vi "PicoLogStart_3.vi"(0 "Ch nr":bool[](array[boolean]), 2 "Single ended\n(0- single)\n(1 - difer)":i32[](array[numeric]) min=0 max=1 step=1, 3 "sampleInterval_ms":i32=1000, 4 "Voltage range":i32[](array[numeric]) min=0 max=6 step=1, 6 "conversionTime":i16(ring) items=["60 ms", "100 ms", "180 ms", "340 ms", "660 ms"], 7 "Mains Frequency":i16(ring) items=["50 Hz", "60 Hz"]) -> (1 "Voltage range":i32[](array[numeric]), 5 "noOfChannels":i16=2, 8 "ChNrSkArr":i32[](array[numeric]), 9 "handle":i16, 10 "STOP":bool)   [LabVIEW 2014]
uses:
  Instance           1 22Saved   HRDL_streaming .vi
  Instance         138 22Saved   HRDL_streaming .vi
  picohrdl.dll
panel:
  out "Unit Info":T1
  # "1       2       3      4       5        6       7       8       9      10     11      12     13    14       15     16"
  # "0 -+2500mV\n1 -+1250mV\n2 -+625mV\n3 -+313mV\n4 -+156mV\n5 -+78mv\n6 -+39mV"
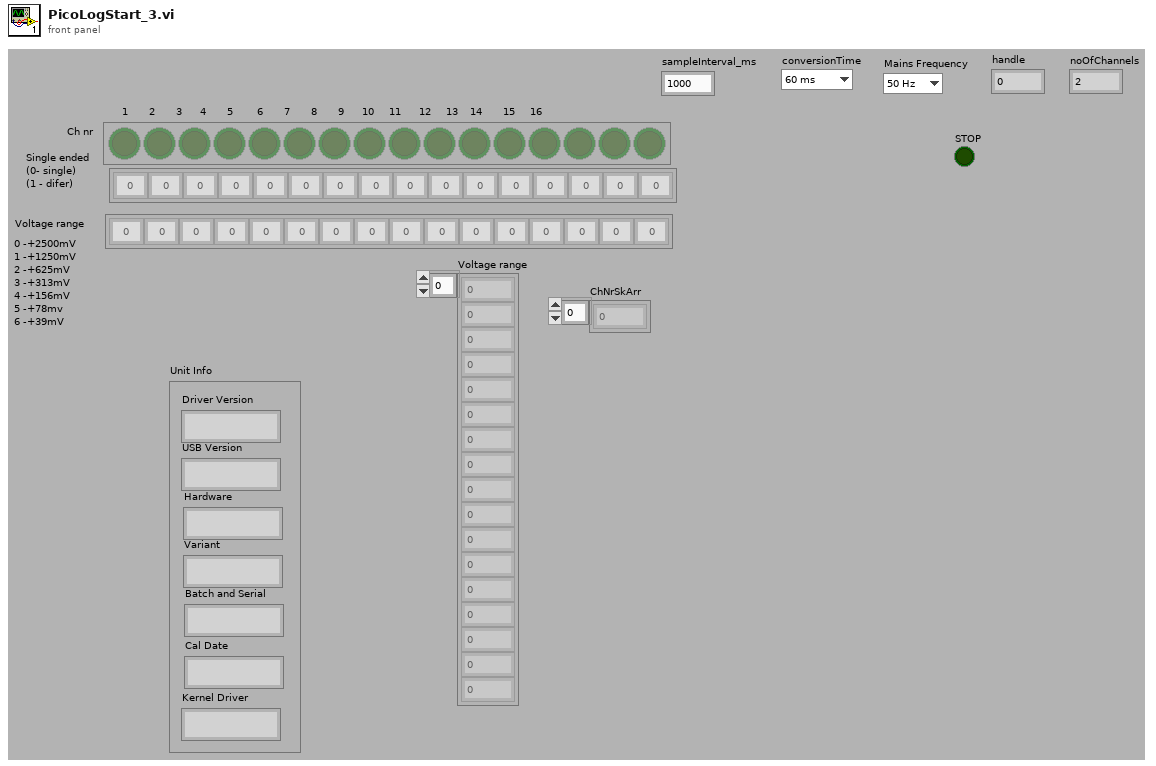
[diagram p1: front panel]
types:
  T1 = cluster{"Driver Version":string, "USB Version":string, "Hardware":string, "Variant":string, "Batch and Serial":string, "Cal Date":string, "Kernel Driver":string}
  T2 = cluster{"[0]":string, "[1]":string, "[2]":string, "[3]":string, "[4]":string, "[5]":string, "[6]":string}
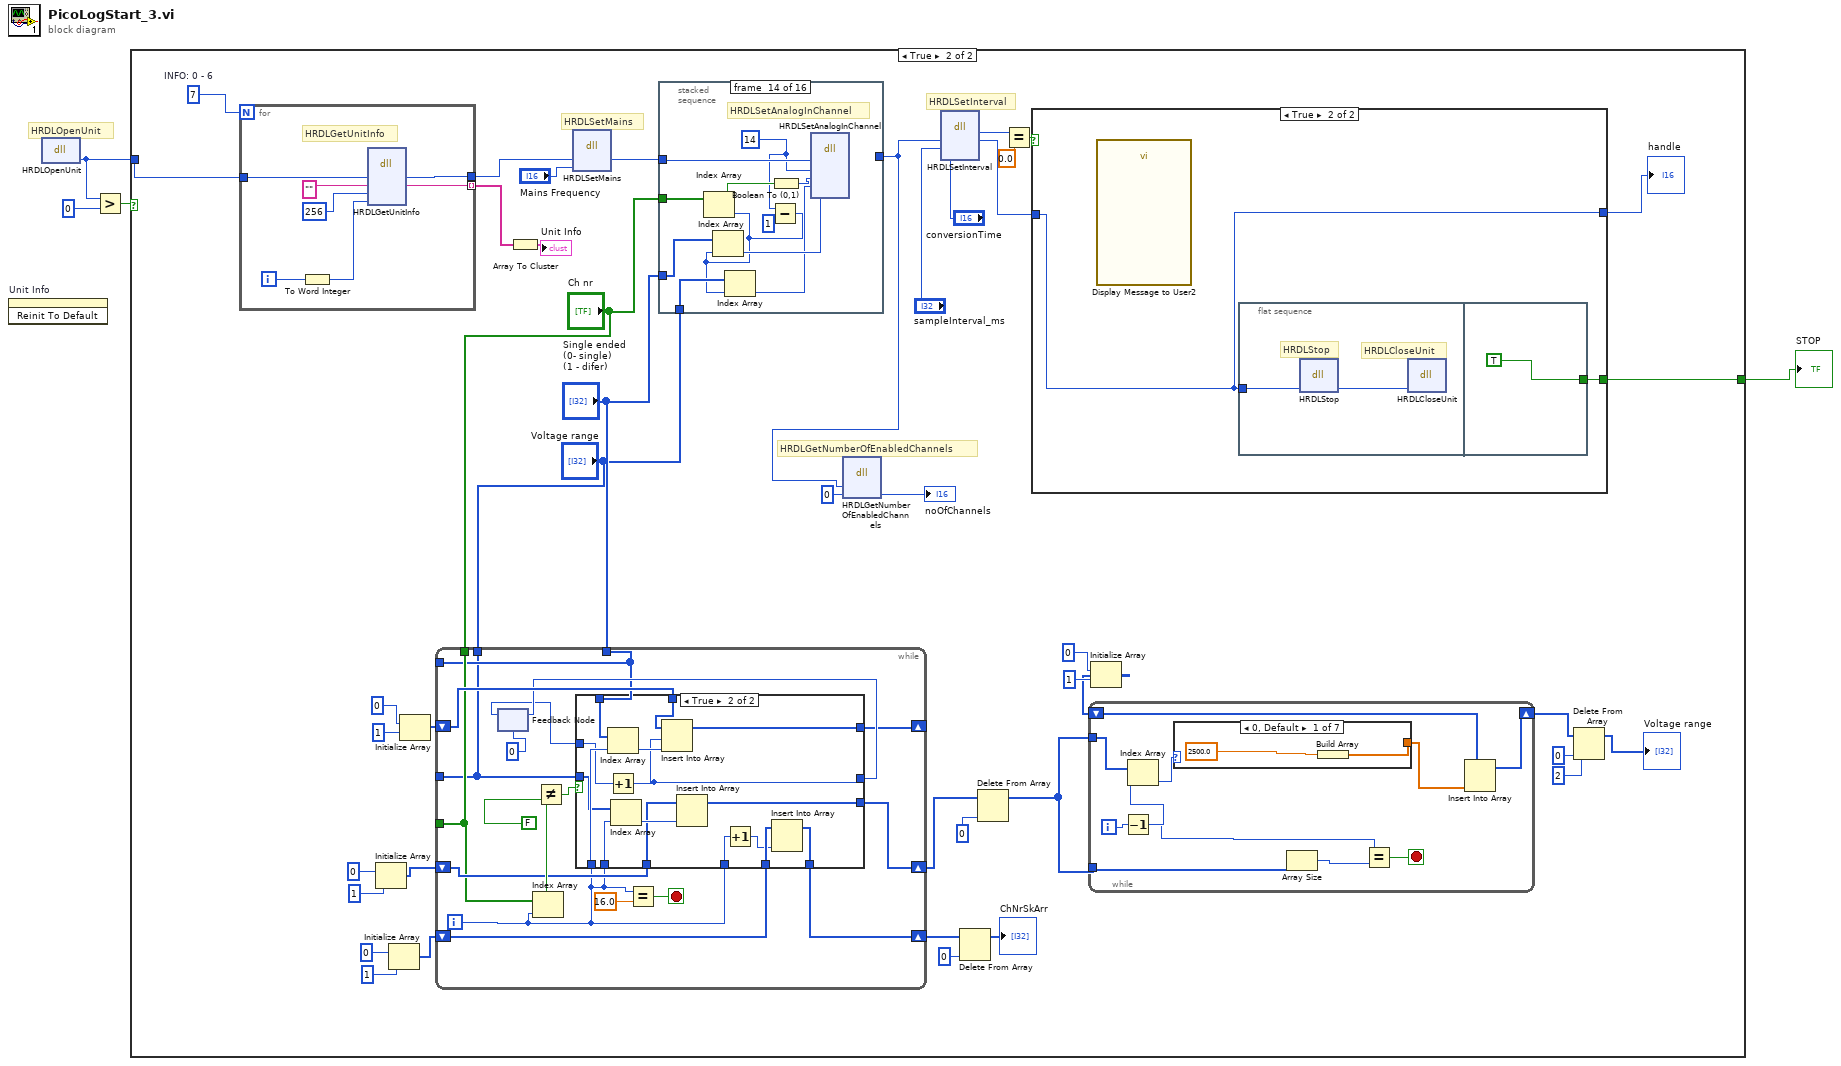
[diagram p0: block diagram]
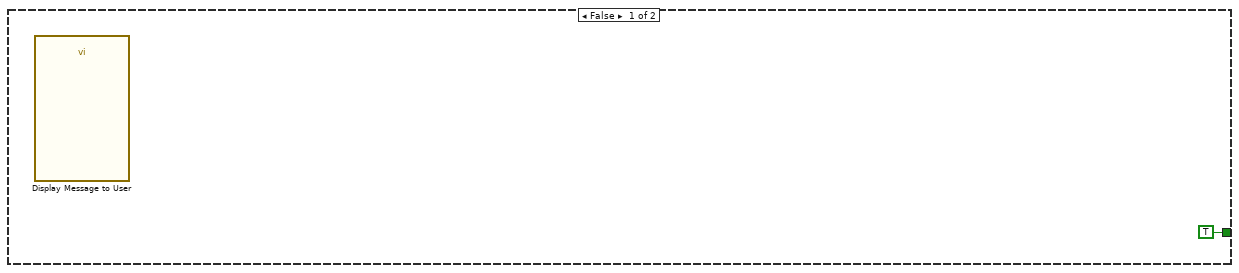
[diagram p2: hidden frame]
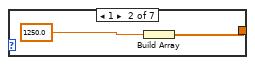
[diagram p3: hidden frame]
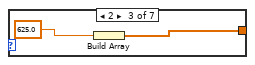
[diagram p4: hidden frame]
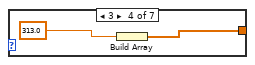
[diagram p5: hidden frame]
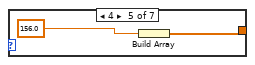
[diagram p6: hidden frame]
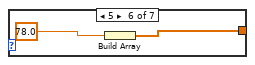
[diagram p7: hidden frame]
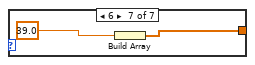
[diagram p8: hidden frame]
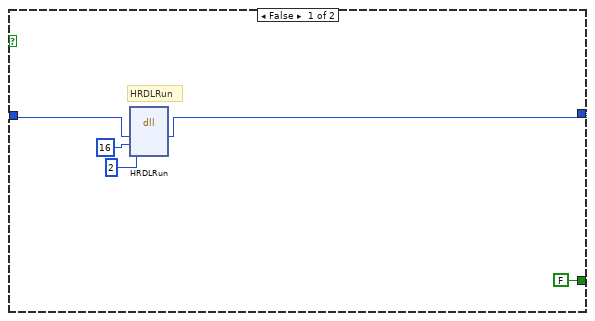
[diagram p10: hidden frame]
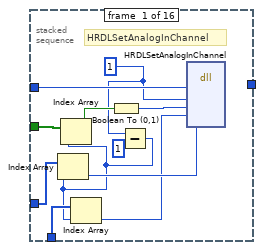
[diagram p11: hidden frame]
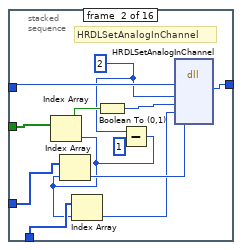
[diagram p12: hidden frame]
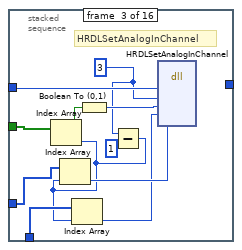
[diagram p13: hidden frame]
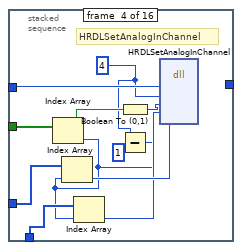
[diagram p14: hidden frame]
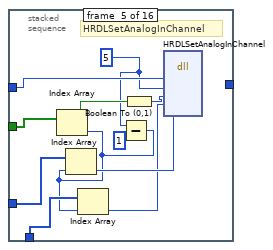
[diagram p15: hidden frame]
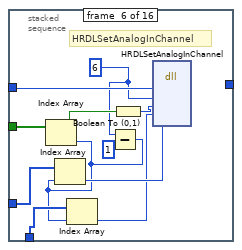
[diagram p16: hidden frame]
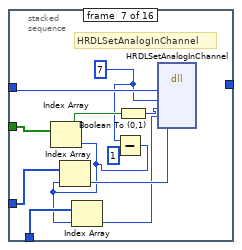
[diagram p17: hidden frame]
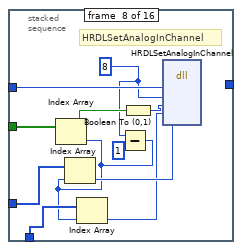
[diagram p18: hidden frame]
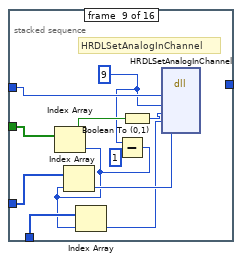
[diagram p19: hidden frame]
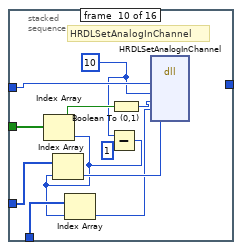
[diagram p20: hidden frame]
diagram:
  # "HRDLOpenUnit"
  n1 = invoke on="Unit Info" class="Clust (strict)" method="Reinit To Default"() -> ()  [unwired: 3 in, 3 out]
  n2 = dll-call lib="picohrdl.dll" fn="HRDLOpenUnit"() -> ("handle"=w2:i16)  [unwired: 3 in, 2 out]
  n3 = Greater?(x=w2, y=i16 0) -> (0:w4:bool)
  n4 = case shown="True" w4 {
    tunnel: w2 -> [_ w39]
    tunnel: [TRUE ("stop") w33] -> w1
    frame False {
      n5 = call "Display Message to User"() -> ()  [unwired: 10 in, 2 out]
    }
    frame True {
      w41 = 7  # INFO: 0 - 6
      # "HRDLGetNumberOfEnabledChannels"
      # "HRDLSetInterval"
      # "HRDLSetMains"
      n6 = for {
        N: w41 -> [_]
        tunnel: w39 -> [w117]
        tunnel: [w114] -> w38 mode=indexing
        tunnel: [w112] -> w40
        i -> [w113]
        # "HRDLGetUnitInfo"
        n7 = To Word Integer(number=w113) -> (16bit integer=w111:i16)
        n8 = dll-call lib="picohrdl.dll" fn="HRDLGetUnitInfo"("handle"=w117, "unitInfo"="", "stringLength"=i16 256, "info"=w111) -> ("handle"=w112:i16, "unitInfo"=w114:string)  [unwired: 6 in, 2 out]
      }
      n9 = Initialize Array(0 ("element"), 1 ("dimension size")) -> (w28:i32[])
      n10 = Initialize Array(0 ("element"), 1 ("dimension size")) -> (w9:i32[])
      n11 = Initialize Array(0 ("element"), 1 ("dimension size")) -> (w25:i32[])
      n12 = while {
        tunnel: [w78] -> _
        tunnel: [w77] -> _
        tunnel: [w76] -> _
        shift-right: [w82] -> w23
        shift-left: w28 -> [w81]
        shift-right: [w80] -> _
        shift-left: w25 -> [w87]
        tunnel: "Ch nr" -> [w78]
        tunnel: "Single ended\n(0- single)\n(1 - difer)" -> [w77]
        tunnel: "Voltage range" -> [w76]
        shift-right: [w73] -> w8
        shift-left: w9 -> [w75]
        i -> [w74]
        stop <- w83 stop-if-true
        n13 = feedback #1(i16 0 ("handle")) -> (w79:i16)
        n14 = Index Array(array=w78, index=w74) -> (element=w90:bool)
        n15 = Not Equal?(x=w90, y=FALSE) -> (x != y?=w88:bool)
        n16 = case shown="True" w88 {
          tunnel: w77 -> [_ w109]
          tunnel: w74 -> [_ w110]
          tunnel: w87 -> [w92 w107]
          tunnel: w79 -> [w94 w106]
          tunnel: [w94 w102] -> w85
          tunnel: w74 -> [_ w105]
          tunnel: w76 -> [_ w104]
          tunnel: [w93 w101] -> w82
          tunnel: w81 -> [w93 w100]
          tunnel: [w92 w99] -> w80
          tunnel: w75 -> [w91 w98]
          tunnel: w74 -> [_ w96]
          tunnel: [w91 w95] -> w73
          frame False {
          }
          frame True {
            n17 = Index Array(array=w109, index=w110) -> (element=w108:i32)
            n18 = Increment(x=w106) -> (x+1=w102:i16)
            n19 = Index Array(array=w104, index=w105) -> (element=w103:i32)
            n20 = Insert Into Array(array=w107, index=w102, new element=w108) -> (w99:i32[])
            n21 = Insert Into Array(array=w100, new element=w103) -> (w101:i32[])  [unwired: 1 in]
            n22 = Increment(x=w96) -> (x+1=w97:i32)
            n23 = Insert Into Array(array=w98, new element=w97) -> (w95:i32[])  [unwired: 1 in]
          }
        }
        n24 = feedback-in #1(w85) -> ()
        n25 = Equal?(x=w74, y=16.0) -> (x = y?=w83:bool)
      }
      n26 = Array To Cluster(array=w38) -> (cluster=→"Unit Info":T2)
      n27 = dll-call lib="PicoHRDL.dll" fn="HRDLSetMains"("handle"=w40, "sixtyHertz"="Mains Frequency") -> ("handle"=w32:i16)  [unwired: 5 in, 2 out]
      n28 = stacked-sequence {
        tunnel: w32 -> [w138 w146 w157 w165 w179 w190 w201 w212 w223 w234 w245 w256 w267 w278 w289 w300]
        tunnel: "Ch nr" -> [w136 w145 w156 w168 w178 w189 w200 w211 w222 w233 w244 w255 w266 w277 w288 w299]
        tunnel: "Single ended\n(0- single)\n(1 - difer)" -> [w134 w144 w155 w166 w177 w188 w199 w210 w221 w232 w243 w254 w265 w276 w287 w298]
        tunnel: "Voltage range" -> [w132 w143 w154 w167 w176 w187 w198 w209 w220 w231 w242 w253 w264 w275 w286 w297]
        tunnel: [_ w139 _ _ _ _ _ _ _ _ _ _ _ _ _ _] -> w31
        frame #0 {
          w130 = i16 1 ("channel")
          # "HRDLSetAnalogInChannel"
          n29 = Subtract(x=w130, y=i16 1) -> (x-y=w129:i16)
          n30 = Index Array(array=w134, index=w129) -> (element=w133:i32)
          n31 = Index Array(array=w136, index=w129) -> (element=w135:bool)
          n32 = Index Array(array=w132, index=w129) -> (element=w131:i32)
          n33 = Boolean To (0,1)(Boolean=w135) -> (0, 1=w137:i16)
          n34 = dll-call lib="PicoHRDL.dll" fn="HRDLSetAnalogInChannel"("handle"=w138, "channel"=w130, "enabled"=w137, "range"=w131, "singleEnded"=w133) -> ()  [unwired: 9 in, 2 out]
        }
        frame #1 {
          w141 = i16 2 ("channel")
          # "HRDLSetAnalogInChannel"
          n35 = Subtract(x=w141, y=i16 1) -> (x-y=w140:i16)
          n36 = Index Array(array=w145, index=w140) -> (element=w149:bool)
          n37 = Index Array(array=w144, index=w140) -> (element=w148:i32)
          n38 = Index Array(array=w143, index=w140) -> (element=w147:i32)
          n39 = Boolean To (0,1)(Boolean=w149) -> (0, 1=w150:i16)
          n40 = dll-call lib="PicoHRDL.dll" fn="HRDLSetAnalogInChannel"("handle"=w146, "channel"=w141, "enabled"=w150, "range"=w147, "singleEnded"=w148) -> ("handle"=w139:i16)  [unwired: 8 in, 2 out]
        }
        frame #2 {
          w152 = i16 3 ("channel")
          # "HRDLSetAnalogInChannel"
          n41 = Subtract(x=w152, y=i16 1) -> (x-y=w151:i16)
          n42 = Index Array(array=w156, index=w151) -> (element=w160:bool)
          n43 = Index Array(array=w155, index=w151) -> (element=w159:i32)
          n44 = Index Array(array=w154, index=w151) -> (element=w158:i32)
          n45 = Boolean To (0,1)(Boolean=w160) -> (0, 1=w161:i16)
          n46 = dll-call lib="PicoHRDL.dll" fn="HRDLSetAnalogInChannel"("handle"=w157, "channel"=w152, "enabled"=w161, "range"=w158, "singleEnded"=w159) -> ()  [unwired: 9 in, 2 out]
        }
        frame #3 {
          w163 = i16 4 ("channel")
          # "HRDLSetAnalogInChannel"
          n47 = Subtract(x=w163, y=i16 1) -> (x-y=w162:i16)
          n48 = Index Array(array=w168, index=w162) -> (element=w171:bool)
          n49 = Index Array(array=w166, index=w162) -> (element=w170:i32)
          n50 = Index Array(array=w167, index=w162) -> (element=w169:i32)
          n51 = Boolean To (0,1)(Boolean=w171) -> (0, 1=w172:i16)
          n52 = dll-call lib="PicoHRDL.dll" fn="HRDLSetAnalogInChannel"("handle"=w165, "channel"=w163, "enabled"=w172, "range"=w169, "singleEnded"=w170) -> ()  [unwired: 9 in, 2 out]
        }
        frame #4 {
          w174 = i16 5 ("channel")
          # "HRDLSetAnalogInChannel"
          n53 = Subtract(x=w174, y=i16 1) -> (x-y=w173:i16)
          n54 = Index Array(array=w178, index=w173) -> (element=w182:bool)
          n55 = Index Array(array=w177, index=w173) -> (element=w181:i32)
          n56 = Index Array(array=w176, index=w173) -> (element=w180:i32)
          n57 = Boolean To (0,1)(Boolean=w182) -> (0, 1=w183:i16)
          n58 = dll-call lib="PicoHRDL.dll" fn="HRDLSetAnalogInChannel"("handle"=w179, "channel"=w174, "enabled"=w183, "range"=w180, "singleEnded"=w181) -> ()  [unwired: 9 in, 2 out]
        }
        frame #5 {
          w185 = i16 6 ("channel")
          # "HRDLSetAnalogInChannel"
          n59 = Subtract(x=w185, y=i16 1) -> (x-y=w184:i16)
          n60 = Index Array(array=w189, index=w184) -> (element=w193:bool)
          n61 = Index Array(array=w188, index=w184) -> (element=w192:i32)
          n62 = Index Array(array=w187, index=w184) -> (element=w191:i32)
          n63 = Boolean To (0,1)(Boolean=w193) -> (0, 1=w194:i16)
          n64 = dll-call lib="PicoHRDL.dll" fn="HRDLSetAnalogInChannel"("handle"=w190, "channel"=w185, "enabled"=w194, "range"=w191, "singleEnded"=w192) -> ()  [unwired: 9 in, 2 out]
        }
        frame #6 {
          w196 = i16 7 ("channel")
          # "HRDLSetAnalogInChannel"
          n65 = Subtract(x=w196, y=i16 1) -> (x-y=w195:i16)
          n66 = Index Array(array=w200, index=w195) -> (element=w204:bool)
          n67 = Index Array(array=w199, index=w195) -> (element=w203:i32)
          n68 = Index Array(array=w198, index=w195) -> (element=w202:i32)
          n69 = Boolean To (0,1)(Boolean=w204) -> (0, 1=w205:i16)
          n70 = dll-call lib="PicoHRDL.dll" fn="HRDLSetAnalogInChannel"("handle"=w201, "channel"=w196, "enabled"=w205, "range"=w202, "singleEnded"=w203) -> ()  [unwired: 9 in, 2 out]
        }
        frame #7 {
          w207 = i16 8 ("channel")
          # "HRDLSetAnalogInChannel"
          n71 = Subtract(x=w207, y=i16 1) -> (x-y=w206:i16)
          n72 = Index Array(array=w211, index=w206) -> (element=w215:bool)
          n73 = Index Array(array=w210, index=w206) -> (element=w214:i32)
          n74 = Index Array(array=w209, index=w206) -> (element=w213:i32)
          n75 = Boolean To (0,1)(Boolean=w215) -> (0, 1=w216:i16)
          n76 = dll-call lib="PicoHRDL.dll" fn="HRDLSetAnalogInChannel"("handle"=w212, "channel"=w207, "enabled"=w216, "range"=w213, "singleEnded"=w214) -> ()  [unwired: 9 in, 2 out]
        }
        frame #8 {
          w218 = i16 9 ("channel")
          # "HRDLSetAnalogInChannel"
          n77 = Subtract(x=w218, y=i16 1) -> (x-y=w217:i16)
          n78 = Index Array(array=w222, index=w217) -> (element=w226:bool)
          n79 = Index Array(array=w221, index=w217) -> (element=w225:i32)
          n80 = Index Array(array=w220, index=w217) -> (element=w224:i32)
          n81 = Boolean To (0,1)(Boolean=w226) -> (0, 1=w227:i16)
          n82 = dll-call lib="PicoHRDL.dll" fn="HRDLSetAnalogInChannel"("handle"=w223, "channel"=w218, "enabled"=w227, "range"=w224, "singleEnded"=w225) -> ()  [unwired: 9 in, 2 out]
        }
        frame #9 {
          w229 = i16 10 ("channel")
          # "HRDLSetAnalogInChannel"
          n83 = Subtract(x=w229, y=i16 1) -> (x-y=w228:i16)
          n84 = Index Array(array=w233, index=w228) -> (element=w237:bool)
          n85 = Index Array(array=w232, index=w228) -> (element=w236:i32)
          n86 = Index Array(array=w231, index=w228) -> (element=w235:i32)
          n87 = Boolean To (0,1)(Boolean=w237) -> (0, 1=w238:i16)
          n88 = dll-call lib="PicoHRDL.dll" fn="HRDLSetAnalogInChannel"("handle"=w234, "channel"=w229, "enabled"=w238, "range"=w235, "singleEnded"=w236) -> ()  [unwired: 9 in, 2 out]
        }
        frame #10 {
          w240 = i16 11 ("channel")
          # "HRDLSetAnalogInChannel"
          n89 = Subtract(x=w240, y=i16 1) -> (x-y=w239:i16)
          n90 = Index Array(array=w244, index=w239) -> (element=w248:bool)
          n91 = Index Array(array=w243, index=w239) -> (element=w247:i32)
          n92 = Index Array(array=w242, index=w239) -> (element=w246:i32)
          n93 = Boolean To (0,1)(Boolean=w248) -> (0, 1=w249:i16)
          n94 = dll-call lib="PicoHRDL.dll" fn="HRDLSetAnalogInChannel"("handle"=w245, "channel"=w240, "enabled"=w249, "range"=w246, "singleEnded"=w247) -> ()  [unwired: 9 in, 2 out]
        }
        frame #11 {
          w251 = i16 12 ("channel")
          # "HRDLSetAnalogInChannel"
          n95 = Subtract(x=w251, y=i16 1) -> (x-y=w250:i16)
          n96 = Index Array(array=w255, index=w250) -> (element=w259:bool)
          n97 = Index Array(array=w254, index=w250) -> (element=w258:i32)
          n98 = Index Array(array=w253, index=w250) -> (element=w257:i32)
          n99 = Boolean To (0,1)(Boolean=w259) -> (0, 1=w260:i16)
          n100 = dll-call lib="PicoHRDL.dll" fn="HRDLSetAnalogInChannel"("handle"=w256, "channel"=w251, "enabled"=w260, "range"=w257, "singleEnded"=w258) -> ()  [unwired: 9 in, 2 out]
        }
        frame #12 {
          w262 = i16 13 ("channel")
          # "HRDLSetAnalogInChannel"
          n101 = Subtract(x=w262, y=i16 1) -> (x-y=w261:i16)
          n102 = Index Array(array=w266, index=w261) -> (element=w270:bool)
          n103 = Index Array(array=w265, index=w261) -> (element=w269:i32)
          n104 = Index Array(array=w264, index=w261) -> (element=w268:i32)
          n105 = Boolean To (0,1)(Boolean=w270) -> (0, 1=w271:i16)
          n106 = dll-call lib="PicoHRDL.dll" fn="HRDLSetAnalogInChannel"("handle"=w267, "channel"=w262, "enabled"=w271, "range"=w268, "singleEnded"=w269) -> ()  [unwired: 9 in, 2 out]
        }
        frame #13 {
          w273 = i16 14 ("channel")
          # "HRDLSetAnalogInChannel"
          n107 = Subtract(x=w273, y=i16 1) -> (x-y=w272:i16)
          n108 = Index Array(array=w277, index=w272) -> (element=w281:bool)
          n109 = Index Array(array=w276, index=w272) -> (element=w280:i32)
          n110 = Index Array(array=w275, index=w272) -> (element=w279:i32)
          n111 = Boolean To (0,1)(Boolean=w281) -> (0, 1=w282:i16)
          n112 = dll-call lib="PicoHRDL.dll" fn="HRDLSetAnalogInChannel"("handle"=w278, "channel"=w273, "enabled"=w282, "range"=w279, "singleEnded"=w280) -> ()  [unwired: 9 in, 2 out]
        }
        frame #14 {
          w284 = i16 15 ("channel")
          # "HRDLSetAnalogInChannel"
          n113 = Subtract(x=w284, y=i16 1) -> (x-y=w283:i16)
          n114 = Index Array(array=w288, index=w283) -> (element=w292:bool)
          n115 = Index Array(array=w287, index=w283) -> (element=w291:i32)
          n116 = Index Array(array=w286, index=w283) -> (element=w290:i32)
          n117 = Boolean To (0,1)(Boolean=w292) -> (0, 1=w293:i16)
          n118 = dll-call lib="PicoHRDL.dll" fn="HRDLSetAnalogInChannel"("handle"=w289, "channel"=w284, "enabled"=w293, "range"=w290, "singleEnded"=w291) -> ()  [unwired: 9 in, 2 out]
        }
        frame #15 {
          w295 = i16 16 ("channel")
          # "HRDLSetAnalogInChannel"
          n119 = Subtract(x=w295, y=i16 1) -> (x-y=w294:i16)
          n120 = Index Array(array=w299, index=w294) -> (element=w303:bool)
          n121 = Index Array(array=w298, index=w294) -> (element=w302:i32)
          n122 = Index Array(array=w297, index=w294) -> (element=w301:i32)
          n123 = Boolean To (0,1)(Boolean=w303) -> (0, 1=w304:i16)
          n124 = dll-call lib="PicoHRDL.dll" fn="HRDLSetAnalogInChannel"("handle"=w300, "channel"=w295, "enabled"=w304, "range"=w301, "singleEnded"=w302) -> ()  [unwired: 9 in, 2 out]
        }
      }
      n125 = dll-call lib="PicoHRDL.dll" fn="HRDLGetNumberOfEnabledChannels"("handle"=w31, "nEnabledChannels"=i16 0) -> ("nEnabledChannels"=→"noOfChannels":i16)  [unwired: 5 in, 2 out]
      n126 = dll-call lib="PicoHRDL.dll" fn="HRDLSetInterval"("handle"=w31, "sampleInterval_ms"="sampleInterval_ms", "conversionTime"="conversionTime") -> ("return type"=w45:i16, "handle"=w44:i16)  [unwired: 5 in, 2 out]
      n127 = Delete From Array(array=w8, index=0) -> (array with subset deleted=→"ChNrSkArr":i32[])  [unwired: 1 in, 1 out]
      n128 = Delete From Array(array=w23, index=0 ("length")) -> (array with subset deleted=w15:i32[])  [unwired: 1 in, 1 out]
      n129 = Equal?(x=w45, y=0.0) -> (x = y?=w43:bool)
      n130 = case shown="True" w43 {
        tunnel: [w119 w124] -> w36
        tunnel: w44 -> [w120 w124]
        tunnel: [FALSE ("stop") w123] -> w33
        frame False {
          # "HRDLRun"
          n131 = dll-call lib="PicoHRDL.dll" fn="HRDLRun"("handle"=w120, "nValues"=16, "method"=i16 2) -> ("handle"=w119:i16)  [unwired: 6 in, 2 out]
        }
        frame True {
          n132 = call "Display Message to User2"() -> ()  [unwired: 10 in, 2 out]
          n133 = flat-sequence {
            tunnel: w124 -> [w125]
            tunnel: [TRUE ("stop")] -> w123
            frame #0 {
              # "HRDLStop"
              # "HRDLCloseUnit"
              n134 = dll-call lib="picohrdl.dll" fn="HRDLStop"("handle"=w125) -> ("handle"=w126:i16)  [unwired: 4 in, 2 out]
              n135 = dll-call lib="PicoHRDL.dll" fn="HRDLCloseUnit"("handle"=w126) -> ()  [unwired: 5 in, 2 out]
            }
            frame #1 {
            }
          }
        }
      }
      "handle" <- w36
      n136 = Initialize Array(0 ("element"), 1 ("dimension size")) -> (w20:i32[])
      n137 = while {
        tunnel: w15 -> [w58]
        tunnel: w15 -> [w54]
        shift-right: [w50] -> w17
        shift-left: w20 -> [w53]
        i -> [w49]
        stop <- w55 stop-if-true
        n138 = Decrement(x=w49) -> (x-1=w52:i32)
        n139 = Index Array(array=w58, index=w52) -> (element=w57:i32)
        n140 = case shown="0, Default" w57 {
          tunnel: [w59 w61 w63 w65 w67 w69 w71] -> w51
          frame 0, Default {
            n141 = Build Array(2500.0 ("element")) -> (w59:dbl[])
          }
          frame 1 {
            n142 = Build Array(1250.0 ("element")) -> (w61:dbl[])
          }
          frame 2 {
            n143 = Build Array(625.0 ("element")) -> (w63:dbl[])
          }
          frame 3 {
            n144 = Build Array(313.0 ("element")) -> (w65:dbl[])
          }
          frame 4 {
            n145 = Build Array(156.0 ("element")) -> (w67:dbl[])
          }
          frame 5 {
            n146 = Build Array(78.0 ("element")) -> (w69:dbl[])
          }
          frame 6 {
            n147 = Build Array(39.0 ("element")) -> (w71:dbl[])
          }
        }
        n148 = Array Size(array=w54) -> (size(s)=w56:i32)
        n149 = Equal?(x=w49, y=w56) -> (x = y?=w55:bool)
        n150 = Insert Into Array(array=w53, new element=w51) -> (w50:i32[])  [unwired: 1 in]
      }
      n151 = Delete From Array(array=w17, length=2, index=0) -> (array with subset deleted=→"Voltage range":i32[])  [unwired: 1 out]
    }
  }
  "STOP" <- w1
